vi "Distance_To_Encoder_Revolutions.vi"(8 "Low Gear?":bool=TRUE, 11 "Target Distance (Feet)":dbl) -> (2 "Target Encoder Value":dbl)   [LabVIEW 2016]
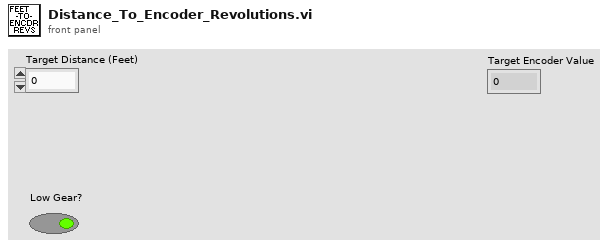
[diagram p1: front panel]
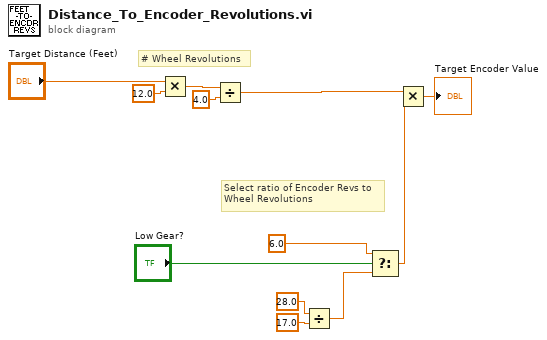
[diagram p0: block diagram]
diagram:
  # "Select ratio of Encoder Revs to\nWheel Revolutions"
  # "# Wheel Revolutions"
  n1 = Multiply(x="Target Distance (Feet)", y=12.0) -> (x*y=w10:dbl)
  n2 = Divide(x=w10, y=4.0) -> (x/y=w3:dbl)
  n3 = Divide(x=28.0, y=17.0) -> (x/y=w4:dbl)
  n4 = Select(t=6.0, s="Low Gear?", f=w4) -> (s? t:f=w2:dbl)
  n5 = Multiply(x=w3, y=w2) -> (x*y=→"Target Encoder Value":dbl)
